vi "Write and Read Holding Registers.vi"(5 "Read Count":u16, 6 "timeout ms (1000)":i32=1000, 7 "Read Start Address":u16, 8 "error in (no error)":errorcluster, 9 "Write Values":u16[](array[numeric]), 10 "Start Address":u16, 11 "Modbus TCP Micro Master in":refnum<class "Modbus TCP Micro Master.lvclass">) -> (0 "error out":errorcluster, 1 "Read Values":u16[](array[numeric]), 3 "Modbus TCP Micro Master out":refnum<class "Modbus TCP Micro Master.lvclass">)   [LabVIEW 2023, in "Modbus TCP Micro.lvlib" / "Modbus TCP Micro Master.lvclass"]
uses:
  Modbus TCP Micro Master.lvclass
  Modbus TCP Micro Master.lvclass/Modbus TCP Micro Master.ctl
  Raw/Modbus Request.vi
  Modbus TCP Micro.lvlib
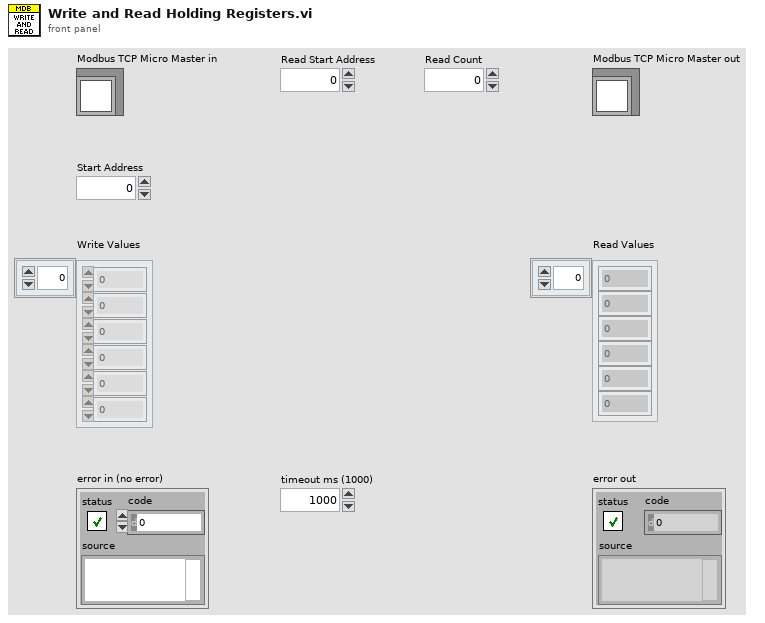
[diagram p1: front panel]
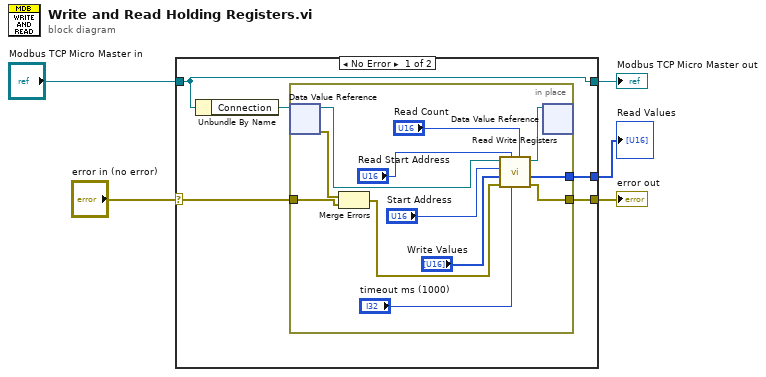
[diagram p0: block diagram]
diagram:
  n1 = case shown="No Error" "error in (no error)" {
    selector: "error in (no error)" -> [w8 w24]
    tunnel: [w7 w24] -> w4
    tunnel: [w10 w23] -> w2
    tunnel: "Modbus TCP Micro Master in" -> [w10 w23]
    tunnel: [w6 _] -> w1
    frame No Error {
      n2 = Unbundle By Name(w10) -> ("Connection"=w9:refnum<data-value>)
      n3 = in-place {
        in-place-border: w8 -> [w22]
        in-place-border: [w21] -> w7
        in-place-border: [w13] -> w6
        n4 = in-place-dvr #1(w9) -> (w18:refnum<k5>, w14:errorcluster)
        n5 = Merge Errors(w14, w22) -> (w15:errorcluster)
        n6 = call "Read Write Registers.vi"("Read Count"="Read Count", "timeout ms (1000)"="timeout ms (1000)", "Read Start Address"="Read Start Address", "error in (no error)"=w15, "Write Values"="Write Values", "Write Start Address"="Start Address", "TCP Network Connection in"=w18) -> ("error out"=w21:errorcluster, "Read Values"=w13:u16[], "TCP Network Connection out"=w17:refnum<k5>)  [unwired: 2 in]
        n7 = in-place-dvr #1(w17) -> ()  [unwired: 2 out]
      }
    }
    frame Error {
    }
  }
  "error out" <- w4
  "Modbus TCP Micro Master out" <- w2
  "Read Values" <- w1
